vi "Detect Freeze.vi"(8 "error in (no error)":errorcluster, 11 "Running image Index":i32) -> (0 "error out":errorcluster)   [LabVIEW 2013]
doc: "Use this template to build a VI to use as a subVI."
uses:
  DB/DbEnum.ctl
  TypeDef/GreyLevelData.ctl
  DB/DisplayGFVEnum.ctl
  DB/DisplayDB.ctl
  <vilib>/vision/Image Controls.llb/IMAQ Image.ctl
  DB/ConfEnum.ctl
  DB/ConfDB.ctl
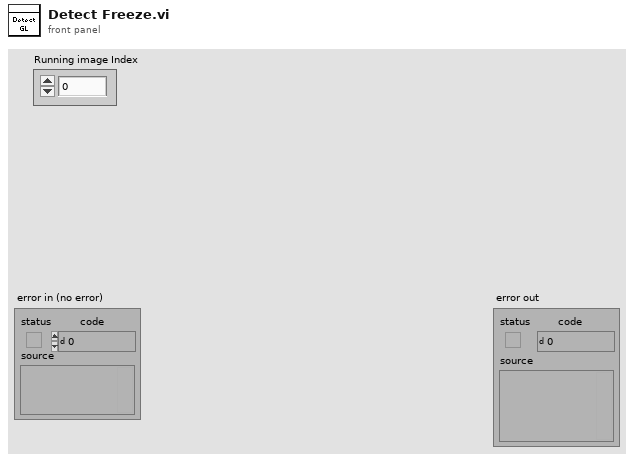
[diagram p1: front panel]
types:
  T1 = typedef "ConfDB.ctl" = cluster{"NumberOfImages":i32, "NoImages2SaveAroundFreeze":i32, "Path":path, "NameOfPartialFile":string, "StartIndex":i32, "NumberOfStdTol":i32, "Detla t (sec)":i32, "Number of images for baseline":i32, "Temperature File Name":string, "Score":dbl, "Index number of Files":i32[], "End Index":i32, "Temperature Array":dbl[], "TStartIndex":i32}
  T2 = typedef "ConfEnum.ctl" = enum16{"Init", "GetConfDB", "GetTemperatureAtIndex", "WriteConfDB", "Configure DB"}
  T3 = typedef "DisplayDB.ctl" = cluster{"Image Ref":T4}
  T4 = typedef "IMAQ Image.ctl" = refnum<image>
  T5 = typedef "DisplayGFVEnum.ctl" = enum16{"Update Display", "Get Image Ref for Analysis", "Insert Image Ref For Analysis", "Insert Image Ref For Display", "Init Display", "Stop Display", "Get Image Ref for Display"}
  T6 = typedef "GreyLevelData.ctl" = cluster{"Grey Level":dbl[], "Grey level diff":dbl[], "ImageIndex":u32, "Drop Index":u32}
  T7 = typedef "DbEnum.ctl" = enum16{"Write DropletDB", "Init", "Insert Detection Result Data", "Insert Grey Level Result", "Insert Baseline Results", "AddFreezeImagesAtCertainDroplet", "UpdateIncludeDroplet", "Insert Freeze Analysis Results", "GetDropDB", "GetNoFreezedDroplets", "GetGreyLevelAndDiff", "GetGreyLevelatIndexTime", "GetDropletsBoundingBox"}
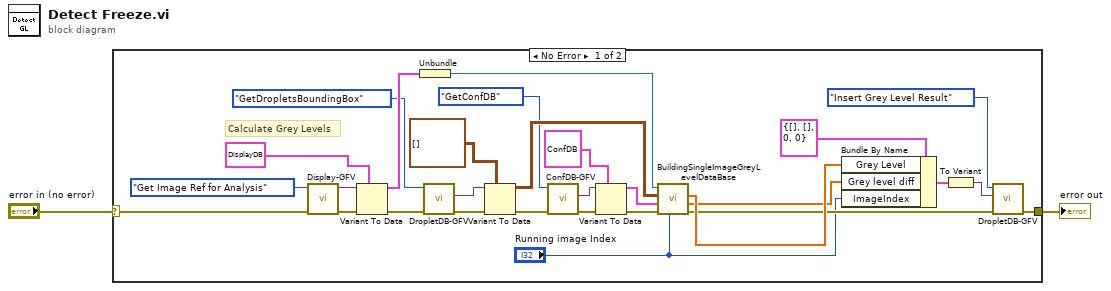
[diagram p0: block diagram]
diagram:
  n1 = case shown="No Error" "error in (no error)" {
    selector: "error in (no error)" -> [w12 w32]
    tunnel: [w3 w32] -> w1
    frame No Error {
      # "Calculate Grey Levels"
      n2 = call "Display-GFV.vi"("error in (no error)"=w12, 11:DisplayGFVEnum."Get Image Ref for Analysis") -> ("error out"=w28:errorcluster, "Data out"=w27:variant)  [unwired: 7 in, 1 out]
      n3 = Variant To Data(error in=w28, type=T3 {"Image Ref"=refnum} ("Display Cluster"), Variant=w27) -> (data=w29:T3, error out=w11:errorcluster)
      n4 = Unbundle(w29) -> ("Image Ref"=w30:T4)
      n5 = call "DropletDB-GFV.vi"("error in (no error)"=w11, "Command In"=DbEnum."GetDropletsBoundingBox") -> ("error out"=w18:errorcluster, "Data out"=w19:variant)  [unwired: 8 in]
      n6 = Variant To Data(error in=w18, type=cluster{"x":sgl, "y":sgl}[][] [] ("Bounding Box"), Variant=w19) -> (data=w31:cluster{"x":sgl, "y":sgl}[][], error out=w10:errorcluster)
      n7 = call "ConfDB-GFV.vi"("error in (no error)"=w10, "Command In"=ConfEnum."GetConfDB") -> ("error out"=w14:errorcluster, "Data out"=w15:variant)  [unwired: 8 in]
      n8 = Variant To Data(error in=w14, type=T1 {"NumberOfImages"=0, "NoImages2SaveAroundFreeze"=0, "Path"=path "", "NameOfPartialFile"="", "StartIndex"=0, "NumberOfStdTol"=0, "Detla t (sec)"=0, "Number of images for baseline"=0, "Temperature File Name"="", "Score"=0.0, "Index number of Files"=[], "End Index"=0, "Temperature Array"=[], "TStartIndex"=0} ("ConfDB"), Variant=w15) -> (data=w5:T1, error out=w9:errorcluster)
      n9 = call "BuildingSingleImageGreyLevelDataBase.vi"("Running Index"="Running image Index", "error in (no error)"=w9, "ConfDB"=w5, "Droplet Bounding Box"=w31, "Image Ref In"=w30) -> ("error out"=w6:errorcluster, "Difference in Grey Level"=w7:dbl[], "GreyLevelArray"=w8:dbl[])  [unwired: 4 in]
      n10 = Bundle By Name(cluster=T6 {"Grey Level"=[], "Grey level diff"=[], "ImageIndex"=0, "Drop Index"=0} ("Cluster"), "Grey Level"=w8, "Grey level diff"=w7, "ImageIndex"="Running image Index") -> (w23:T6)
      n11 = To Variant(anything=w23) -> (Variant=w22:variant)
      n12 = call "DropletDB-GFV.vi"("error in (no error)"=w6, "Data in"=w22, "Command In"=DbEnum."Insert Grey Level Result") -> ("error out"=w3:errorcluster)  [unwired: 7 in, 1 out]
    }
    frame Error {
    }
  }
  "error out" <- w1
